vi "Coeficientes da norma - Não Uniforme.vi"(2 "Tipo de roseta":u16(ring) items=["Roseta A", "Roseta B", "Roseta C"], 3 "Diâmetro do furo":dbl, 4 "Diâmetro da roseta":dbl) -> (0 "Matrizes":T1, 1 "Vetor das medidas":dbl[](array[numeric]))   [LabVIEW 2016]
uses:
  <vilib>/Analysis/baseanly.llb/Real A x B.vi
  <vilib>/Analysis/NI_AALBase.lvlib
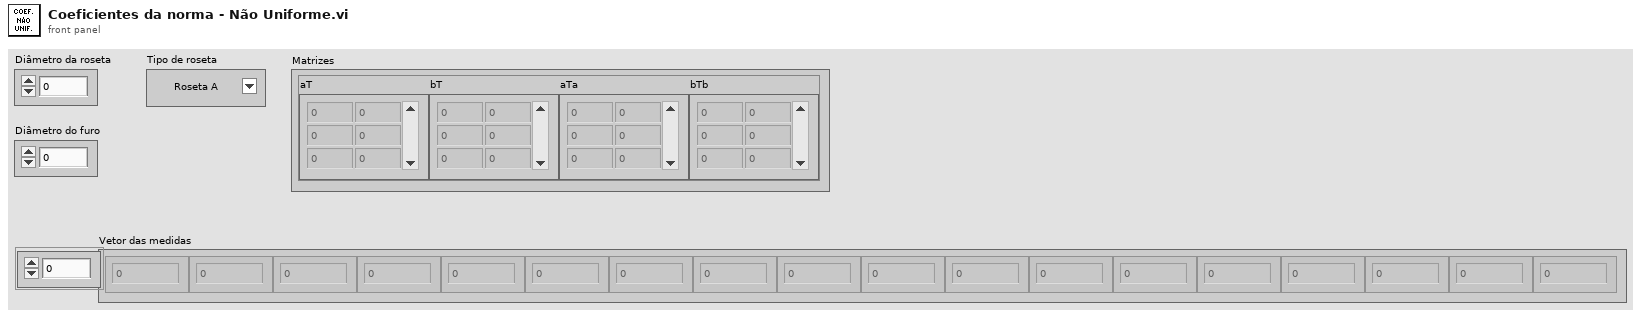
[diagram p1: front panel]
types:
  T1 = typedef "Matrizes não uniforme.ctl" = cluster{"aT":dbl[][], "bT":dbl[][], "aTa":dbl[][], "bTb":dbl[][]}
  T2 = typedef "NI_Matrix.lvlib/RealMatrix.ctl" = dbl[][]
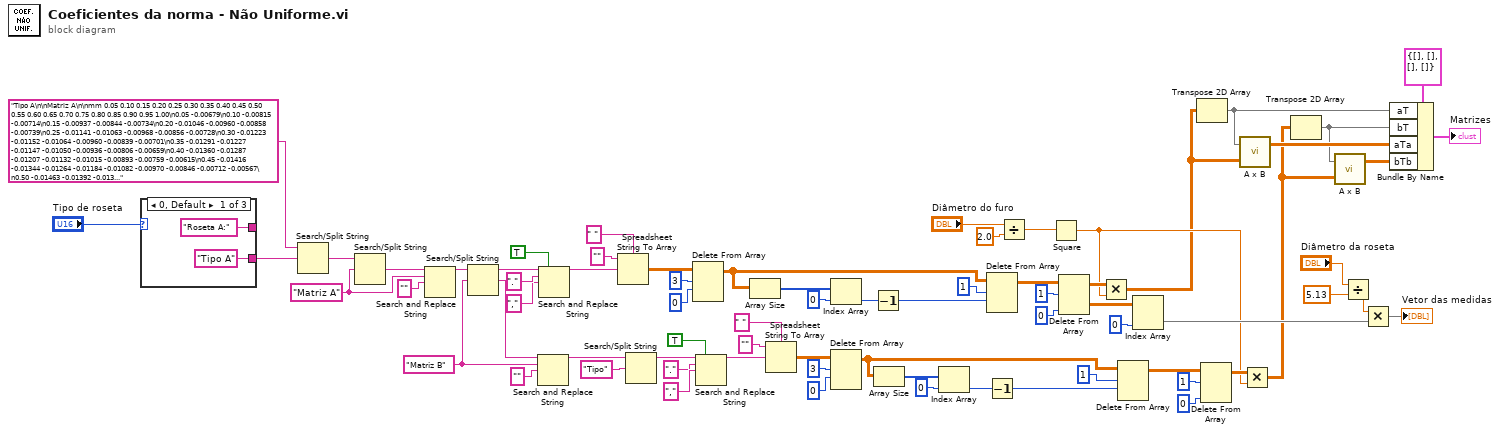
[diagram p0: block diagram]
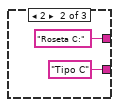
[diagram p2: hidden frame]
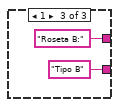
[diagram p3: hidden frame]
diagram:
  w44 = "Matriz B" ("search string/char (-)")
  w69 = "Matriz A" ("search string/char (-)")
  n1 = case shown="0, Default" "Tipo de roseta" {
    tunnel: ["Roseta A:" "Roseta C:" "Roseta B:"] -> _
    tunnel: ["Tipo A" "Tipo C" "Tipo B"] -> w21
    frame 0, Default {
    }
    frame 2 {
    }
    frame 1 {
    }
  }
  n2 = Search/Split String(string="Tipo A\n\nMatriz A\n\nmm 0.05 0.10 0.15 0.20 0.25 0.30 0.35 0.40 0.45 0.50 0.55 0.60 0.65 0.70 0.75 0.80 0.85 0.90 0.95 1.00\n0.05 -0.00679\n0.10 -0.00815 -0.00714\n0.15 -0.00937 -0.00844 -0.00734\n0.20 -0.01046 -0.00960 -0.00858 -0.00739\n0.25 -0.01141 -0.01063 -0.00968 -0.00856 -0.00728\n0.30 -0.01223 -0.01152 -0.01064 -0.00960 -0.00839 -0.00701\n0.35 -0.01291 -0.01227 -0.01147 -0.01050 -0.00936 -0.00806 -0.00659\n0.40 -0.01360 -0.01287 -0.01207 -0.01132 -0.01015 -0.00893 -0.00759 -0.00615\n0.45 -0.01416 -0.01344 -0.01264 -0.01184 -0.01082 -0.00970 -0.00846 -0.00712 -0.00567\n0.50 -0.01463 -0.01392 -0.01312 -0.01223 -0.01134 -0.01031 -0.00917 -0.00793 -0.00657 -0.00511\n0.55 -0.01508 -0.01434 -0.01354 -0.01270 -0.01173 -0.01072 -0.00977 -0.00854 -0.00730 -0.00600 -0.00464\n0.60 -0.01545 -0.01471 -0.01391 -0.01306 -0.01211 -0.01113 -0.01013 -0.00906 -0.00791 -0.00670 -0.00543 -0.00411\n0.65 -0.01578 -0.01503 -0.01422 -0.01340 -0.01243 -0.01146 -0.01049 -0.00938 -0.00842 -0.00722 -0.00604 -0.00485 -0.00364\n0.70 -0.01606 -0.01531 -0.01450 -0.01366 -0.01271 -0.01175 -0.01078 -0.00970 -0.00869 -0.00765 -0.00655 -0.00544 -0.00431 -0.00316\n0.75 -0.01629 -0.01554 -0.01473 -0.01390 -0.01294 -0.01199 -0.01102 -0.00996 -0.00892 -0.00795 -0.00693 -0.00589 -0.00484 -0.00378 -0.00270\n0.80 -0.01649 -0.01574 -0.01493 -0.01410 -0.01313 -0.01217 -0.01123 -0.01018 -0.00919 -0.00815 -0.00716 -0.00624 -0.00524 -0.00425 -0.00328 -0.00231\n0.85 -0.01665 -0.01590 -0.01510 -0.01426 -0.01330 -0.01234 -0.01138 -0.01036 -0.00938 -0.00836 -0.00738 -0.00644 -0.00555 -0.00464 -0.00373 -0.00283 -0.00195\n0.90 -0.01679 -0.01604 -0.01523 -0.01441 -0.01344 -0.01248 -0.01151 -0.01049 -0.00955 -0.00852 -0.00755 -0.00665 -0.00574 -0.00492 -0.00406 -0.00323 -0.00241 -0.00162\n0.95 -0.01692 -0.01617 -0.01536 -0.01452 -0.01357 -0.01261 -0.01164 -0.01063 -0.00967 -0.00866 -0.00770 -0.00679 -0.00592 -0.00508 -0.00432 -0.00353 -0.00277 -0.00203 -0.00131\n1.00 -0.01704 -0.01628 -0.01548 -0.01465 -0.01368 -0.01272 -0.01176 -0.01074 -0.00978 -0.00877 -0.00781 -0.00690 -0.00605 -0.00521 -0.00448 -0.00374 -0.00303 -0.00234 -0.00167 -0.00103\n\nMatriz B\n\nmm 0.05 0.10 0.15 0.20 0.25 0.30 0.35 0.40 0.45 0.50 0.55 0.60 0.65 0.70 0.75 0.80 0.85 0.90 0.95 1.00\n0.05 -0.01264\n0.10 -0.01470 -0.01352\n0.15 -0.01656 -0.01554 -0.01414\n0.20 -0.01821 -0.01735 -0.01611 -0.01449\n0.25 -0.01967 -0.01897 -0.01789 -0.01642 -0.01458\n0.30 -0.02092 -0.02038 -0.01946 -0.01815 -0.01647 -0.01439\n0.35 -0.02197 -0.02159 -0.02083 -0.01968 -0.01815 -0.01624 -0.01395\n0.40 -0.02308 -0.02256 -0.02182 -0.02112 -0.01952 -0.01778 -0.01576 -0.01348\n0.45 -0.02400 -0.02351 -0.02280 -0.02202 -0.02072 -0.01917 -0.01735 -0.01525 -0.01289\n0.50 -0.02481 -0.02434 -0.02366 -0.02273 -0.02167 -0.02031 -0.01868 -0.01678 -0.01460 -0.01216\n0.55 -0.02554 -0.02507 -0.02440 -0.02362 -0.02235 -0.02103 -0.01981 -0.01793 -0.01599 -0.01386 -0.01156\n0.60 -0.02616 -0.02571 -0.02505 -0.02428 -0.02305 -0.02177 -0.02045 -0.01890 -0.01715 -0.01522 -0.01310 -0.01081\n0.65 -0.02668 -0.02625 -0.02561 -0.02487 -0.02364 -0.02239 -0.02109 -0.01949 -0.01813 -0.01623 -0.01430 -0.01226 -0.01013\n0.70 -0.02715 -0.02673 -0.02611 -0.02536 -0.02417 -0.02294 -0.02164 -0.02012 -0.01866 -0.01708 -0.01531 -0.01345 -0.01149 -0.00944\n0.75 -0.02753 -0.02713 -0.02653 -0.02582 -0.02463 -0.02341 -0.02213 -0.02064 -0.01911 -0.01767 -0.01608 -0.01439 -0.01260 -0.01073 -0.00875\n0.80 -0.02789 -0.02749 -0.02690 -0.02620 -0.02502 -0.02382 -0.02256 -0.02108 -0.01968 -0.01807 -0.01652 -0.01511 -0.01344 -0.01172 -0.00995 -0.00812\n0.85 -0.02821 -0.02781 -0.02722 -0.02652 -0.02536 -0.02417 -0.02292 -0.02146 -0.02007 -0.01850 -0.01698 -0.01549 -0.01408 -0.01251 -0.01089 -0.00921 -0.00747\n0.90 -0.02848 -0.02809 -0.02750 -0.02682 -0.02565 -0.02447 -0.02324 -0.02176 -0.02041 -0.01885 -0.01736 -0.01590 -0.01441 -0.01312 -0.011591 -0.01004 -0.00847 -0.00688\n0.95 -0.02871 -0.02832 -0.02774 -0.02706 -0.02591 -0.02473 -0.02350 -0.02204 -0.02067 -0.01916 -0.01769 -0.01624 -0.01480 -0.01340 -0.01213 -0.01072 -0.00928 -0.00781 -0.00632\n1.00 -0.02889 -0.02851 -0.02794 -0.02727 -0.02612 -0.02495 -0.02373 -0.02227 -0.02089 -0.01940 -0.01796 -0.01655 -0.01511 -0.01367 -0.01249 -0.01121 -0.00989 -0.00856 -0.00719 -0.00581\n\nTipo B\n\nMatriz A\n\nmm 0.05 0.10 0.15 0.20 0.25 0.30 0.35 0.40 0.45 0.50 0.55 0.60 0.65 0.70 0.75 0.80 0.85 0.90 0.95 1.00\n0.05 -0.00726\n0.10 -0.00878 -0.00766\n0.15 -0.01013 -0.00909 -0.00788\n0.20 -0.01133 -0.01037 -0.00924 -0.00793\n0.25 -0.01237 -0.01149 -0.01043 -0.00921 -0.00781\n0.30 -0.01325 -0.01245 -0.01147 -0.01033 -0.00901 -0.00751\n0.35 -0.01397 -0.01325 -0.01235 -0.01129 -0.01004 -0.00863 -0.00704\n0.40 -0.01471 -0.01388 -0.01297 -0.01214 -0.01088 -0.00956 -0.00811 -0.00654\n0.45 -0.01533 -0.01450 -0.01360 -0.01268 -0.01161 -0.01039 -0.00904 -0.00758 -0.00599\n0.50 -0.01587 -0.01504 -0.01414 -0.01313 -0.01217 -0.01105 -0.00981 -0.00845 -0.00696 -0.00536\n0.55 -0.01634 -0.01550 -0.01460 -0.01367 -0.01257 -0.01147 -0.01046 -0.00909 -0.00774 -0.00633 -0.00486\n0.60 -0.01672 -0.01589 -0.01500 -0.01406 -0.01299 -0.01190 -0.01082 -0.00964 -0.00839 -0.00708 -0.00572 -0.00430\n0.65 -0.01705 -0.01621 -0.01532 -0.01441 -0.01332 -0.01225 -0.01118 -0.00997 -0.00892 -0.00764 -0.00637 -0.00509 -0.00379\n0.70 -0.01735 -0.01651 -0.01561 -0.01468 -0.01362 -0.01255 -0.01148 -0.01031 -0.00921 -0.00810 -0.00691 -0.00571 -0.00450 -0.00327\n0.75 -0.01759 -0.01675 -0.01586 -0.01493 -0.01387 -0.01280 -0.01174 -0.01059 -0.00945 -0.00840 -0.00730 -0.00619 -0.00506 -0.00392 -0.00277\n0.80 -0.01781 -0.01697 -0.01607 -0.01515 -0.01408 -0.01302 -0.01196 -0.01080 -0.00974 -0.00860 -0.00753 -0.00655 -0.00549 -0.00443 -0.00339 -0.00234\n0.85 -0.01799 -0.01715 -0.01625 -0.01533 -0.01426 -0.01320 -0.01213 -0.01099 -0.00992 -0.00881 -0.00775 -0.00674 -0.00581 -0.00484 -0.00387 -0.00291 -0.00195\n0.90 -0.01814 -0.01730 -0.01640 -0.01550 -0.01441 -0.01334 -0.01229 -0.01114 -0.01008 -0.00897 -0.00793 -0.00695 -0.00598 -0.00514 -0.00423 -0.00333 -0.00246 -0.00162\n0.95 -0.01829 -0.01744 -0.01654 -0.01561 -0.01454 -0.01347 -0.01242 -0.01129 -0.01021 -0.00912 -0.00809 -0.00710 -0.00617 -0.00528 -0.00449 -0.00366 -0.00285 -0.00207 -0.00131\n1.00 -0.01843 -0.01757 -0.01666 -0.01573 -0.01465 -0.01358 -0.01253 -0.01140 -0.01035 -0.00925 -0.00822 -0.00724 -0.00632 -0.00541 -0.00466 -0.00389 -0.00314 -0.00242 -0.00172 -0.00104\n\nMatriz B\n\nmm 0.05 0.10 0.15 0.20 0.25 0.30 0.35 0.40 0.45 0.50 0.55 0.60 0.65 0.70 0.75 0.80 0.85 0.90 0.95 1.00\n0.05 -0.01417\n0.10 -0.01653 -0.01516\n0.15 -0.01866 -0.01746 -0.01585\n0.20 -0.02055 -0.01953 -0.01810 -0.01624\n0.25 -0.02222 -0.02138 -0.02012 -0.01844 -0.01634\n0.30 -0.02365 -0.02299 -0.02190 -0.02040 -0.01848 -0.01614\n0.35 -0.02485 -0.02437 -0.02346 -0.02214 -0.02039 -0.01823 -0.01564\n0.40 -0.02610 -0.02547 -0.02459 -0.02375 -0.02195 -0.01997 -0.01769 -0.01510\n0.45 -0.02715 -0.02656 -0.02571 -0.02479 -0.02331 -0.02154 -0.01947 -0.01709 -0.01440\n0.50 -0.02806 -0.02750 -0.02670 -0.02561 -0.02440 -0.02283 -0.02097 -0.01879 -0.01631 -0.01353\n0.55 -0.02888 -0.02833 -0.02755 -0.02664 -0.02517 -0.02365 -0.02225 -0.02008 -0.01787 -0.01546 -0.01285\n0.60 -0.02958 -0.02906 -0.02830 -0.02740 -0.02598 -0.02450 -0.02298 -0.02119 -0.01919 -0.01699 -0.01460 -0.01202\n0.65 -0.03019 -0.02968 -0.02894 -0.02808 -0.02666 -0.02521 -0.02370 -0.02186 -0.02030 -0.01816 -0.01596 -0.01367 -0.01126\n0.70 -0.03072 -0.03023 -0.02950 -0.02864 -0.02727 -0.02584 -0.02435 -0.02257 -0.02089 -0.01910 -0.01710 -0.01499 -0.01278 -0.01046\n0.75 -0.03116 -0.03068 -0.02998 -0.02914 -0.02778 -0.02638 -0.02491 -0.02316 -0.02139 -0.01976 -0.01795 -0.01603 -0.01401 -0.01188 -0.00964\n0.80 -0.03158 -0.03108 -0.03038 -0.02956 -0.02822 -0.02684 -0.02539 -0.02366 -0.02202 -0.02022 -0.01846 -0.01685 -0.01493 -0.01299 -0.01100 -0.00895\n0.85 -0.03192 -0.03143 -0.03073 -0.02990 -0.02859 -0.02723 -0.02580 -0.02410 -0.02247 -0.02071 -0.01899 -0.01729 -0.01567 -0.01390 -0.01207 -0.01019 -0.00825\n0.90 -0.03221 -0.03173 -0.03104 -0.03022 -0.02891 -0.02756 -0.02616 -0.02444 -0.02287 -0.02112 -0.01942 -0.01779 -0.01608 -0.01459 -0.01288 -0.01115 -0.00940 -0.00762\n0.95 -0.03247 -0.03200 -0.03131 -0.03048 -0.02919 -0.02785 -0.02645 -0.02475 -0.02317 -0.02146 -0.01979 -0.01817 -0.01650 -0.01493 -0.01349 -0.01191 -0.01030 -0.00866 -0.00700\n1.00 -0.03268 -0.03222 -0.03154 -0.03074 -0.02944 -0.02810 -0.02671 -0.02501 -0.02342 -0.02173 -0.02008 -0.01848 -0.01684 -0.01521 -0.01389 -0.01245 -0.01098 -0.00948 -0.00796 -0.00641\n\nTipo C\n\nMatriz A\n\nmm 0.05 0.10 0.15 0.20 0.25 0.30 0.35 0.40 0.45 0.50 0.55 0.60 0.65 0.70 0.75 0.80 0.85 0.90 0.95 1.00 1.05 1.10 1.15 1.20 1.25\n0.05 -0.01704\n0.10 -0.02009 -0.01741\n0.15 -0.02285 -0.02043 -0.01749\n0.20 -0.02531 -0.02315 -0.02047 -0.01730\n0.25 -0.02748 -0.02557 -0.02316 -0.02024 -0.01681\n0.30 -0.02945 -0.02757 -0.02547 -0.02310 -0.01965 -0.01608\n0.35 -0.03124 -0.02938 -0.02730 -0.02526 -0.02212 -0.01885 -0.01523\n0.40 -0.03282 -0.03092 -0.02886 -0.02668 -0.02402 -0.02133 -0.01775 -0.01417\n0.45 -0.03422 -0.03230 -0.03023 -0.02806 -0.02549 -0.02306 -0.01988 -0.01659 -0.01307\n0.50 -0.03545 -0.03347 -0.03137 -0.02921 -0.02669 -0.02422 -0.02148 -0.01867 -0.01521 -0.01192\n0.55 -0.03649 -0.03451 -0.03241 -0.03020 -0.02774 -0.02530 -0.02269 -0.02012 -0.01695 -0.01386 -0.01074\n0.60 -0.03735 -0.03534 -0.03324 -0.03108 -0.02865 -0.02621 -0.02370 -0.02123 -0.01824 -0.01546 -0.01243 -0.00949\n0.65 -0.03810 -0.03609 -0.03399 -0.03178 -0.02942 -0.02700 -0.02448 -0.02212 -0.01926 -0.01661 -0.01385 -0.01110 -0.00835\n0.70 -0.03872 -0.03672 -0.03461 -0.03241 -0.03006 -0.02771 -0.02510 -0.02268 -0.02005 -0.01753 -0.01492 -0.01248 -0.00983 -0.00728\n0.75 -0.03927 -0.03727 -0.03516 -0.03293 -0.03059 -0.02826 -0.02568 -0.02320 -0.02064 -0.01823 -0.01572 -0.01344 -0.01102 -0.00864 -0.00630\n0.80 -0.03972 -0.03772 -0.03563 -0.03343 -0.03101 -0.02869 -0.02615 -0.02371 -0.02117 -0.01877 -0.01633 -0.01408 -0.01185 -0.00978 -0.00753 -0.00540\n0.85 -0.04014 -0.03811 -0.03600 -0.03382 -0.03141 -0.02905 -0.02654 -0.02411 -0.02161 -0.01924 -0.01682 -0.01461 -0.01246 -0.01052 -0.00851 -0.00653 -0.00456\n0.90 -0.04050 -0.03845 -0.03632 -0.03412 -0.03173 -0.02935 -0.02688 -0.02445 -0.02198 -0.01964 -0.01724 -0.01501 -0.01296 -0.01100 -0.00924 -0.00742 -0.00561 -0.00381\n0.95 -0.04083 -0.03874 -0.03658 -0.03436 -0.03199 -0.02960 -0.02712 -0.02477 -0.02230 -0.01996 -0.01756 -0.01540 -0.01334 -0.01142 -0.00968 -0.00810 -0.00639 -0.00476 -0.00317\n1.00 -0.04110 -0.03899 -0.03682 -0.03458 -0.03223 -0.02983 -0.02735 -0.02497 -0.02256 -0.02024 -0.01785 -0.01567 -0.01366 -0.01175 -0.01008 -0.00849 -0.00699 -0.00547 -0.00401 -0.00259\n1.05 -0.04131 -0.03920 -0.03702 -0.03477 -0.03244 -0.03010 -0.02756 -0.02513 -0.02274 -0.02048 -0.01808 -0.01589 -0.01388 -0.01204 -0.01037 -0.00883 -0.00733 -0.00596 -0.00468 -0.00335 -0.00210\n1.10 -0.04149 -0.03938 -0.03720 -0.03493 -0.03262 -0.03028 -0.02775 -0.02531 -0.02290 -0.02064 -0.01828 -0.01609 -0.01410 -0.01224 -0.01062 -0.00909 -0.00765 -0.00631 -0.00511 -0.00392 -0.00278 -0.00168\n1.15 -0.04162 -0.03952 -0.03734 -0.03509 -0.03275 -0.03043 -0.02790 -0.02548 -0.02306 -0.02077 -0.01843 -0.01631 -0.01429 -0.01242 -0.01081 -0.00932 -0.00788 -0.00658 -0.00541 -0.00434 -0.00331 -0.00230 -0.00137\n1.20 -0.04175 -0.03965 -0.03748 -0.03521 -0.03287 -0.03054 -0.02802 -0.02561 -0.02320 -0.02091 -0.01855 -0.01643 -0.01444 -0.01258 -0.01098 -0.00949 -0.00807 -0.00679 -0.00565 -0.00463 -0.00367 -0.00275 -0.00188 -0.00105\n1.25 -0.04188 -0.03977 -0.03759 -0.03535 -0.03298 -0.03061 -0.02811 -0.02572 -0.02330 -0.02103 -0.01865 -0.01652 -0.01455 -0.01271 -0.01111 -0.00964 -0.00822 -0.00695 -0.00581 -0.00485 -0.00393 -0.00304 -0.00227 -0.00151 -0.00076\n\nMatriz B\n\nmm 0.05 0.10 0.15 0.20 0.25 0.30 0.35 0.40 0.45 0.50 0.55 0.60 0.65 0.70 0.75 0.80 0.85 0.90 0.95 1.00 1.05 1.10 1.15 1.20 1.25\n0.05 -0.02533\n0.10 -0.02958 -0.02675\n0.15 -0.03345 -0.03109 -0.02767\n0.20 -0.03693 -0.03504 -0.03209 -0.02808\n0.25 -0.04004 -0.03862 -0.03614 -0.03259 -0.02798\n0.30 -0.04292 -0.04164 -0.03970 -0.03704 -0.03244 -0.02744\n0.35 -0.04555 -0.04439 -0.04258 -0.04050 -0.03641 -0.03194 -0.02670\n0.40 -0.04790 -0.04676 -0.04511 -0.04293 -0.03961 -0.03607 -0.03095 -0.02563\n0.45 -0.05005 -0.04892 -0.04728 -0.04526 -0.04211 -0.03909 -0.03458 -0.02976 -0.02442\n0.50 -0.05200 -0.05084 -0.04918 -0.04711 -0.04419 -0.04115 -0.03730 -0.03340 -0.02817 -0.02304\n0.55 -0.05363 -0.05253 -0.05092 -0.04881 -0.04599 -0.04307 -0.03955 -0.03601 -0.03129 -0.02654 -0.02155\n0.60 -0.05495 -0.05391 -0.05237 -0.05036 -0.04758 -0.04467 -0.04136 -0.03798 -0.03362 -0.02952 -0.02466 -0.01984\n0.65 -0.05614 -0.05513 -0.05362 -0.05164 -0.04893 -0.04609 -0.04280 -0.03962 -0.03548 -0.03163 -0.02733 -0.02289 -0.01827\n0.70 -0.05714 -0.05615 -0.05469 -0.05276 -0.05007 -0.04730 -0.04397 -0.04076 -0.03696 -0.03326 -0.02935 -0.02559 -0.02113 -0.01677\n0.75 -0.05804 -0.05706 -0.05560 -0.05371 -0.05105 -0.04829 -0.04503 -0.04179 -0.03811 -0.03461 -0.03085 -0.02745 -0.02345 -0.01944 -0.01536\n0.80 -0.05882 -0.05782 -0.05635 -0.05448 -0.05186 -0.04915 -0.04590 -0.04273 -0.03912 -0.03565 -0.03202 -0.02862 -0.02506 -0.02168 -0.01784 -0.01406\n0.85 -0.05949 -0.05850 -0.05704 -0.05514 -0.05255 -0.04985 -0.04664 -0.04350 -0.03996 -0.03657 -0.03300 -0.02966 -0.02624 -0.02314 -0.1978 -0.01633 -0.01275\n0.90 -0.06006 -0.05908 -0.05762 -0.05571 -0.05315 -0.05044 -0.04727 -0.04412 -0.04068 -0.03734 -0.03382 -0.03048 -0.02723 -0.02407 -0.02126 -0.01813 -0.01487 -0.01149\n0.95 -0.06051 -0.05955 -0.05811 -0.05622 -0.05364 -0.05100 -0.04781 -0.04465 -0.04125 -0.03799 -0.03448 -0.03124 -0.02799 -0.02494 -0.02211 -0.01956 -0.01647 -0.01341 -0.01034\n1.00 -0.06091 -0.05997 -0.05854 -0.05664 -0.05407 -0.05142 -0.04828 -0.04513 -0.04176 -0.03850 -0.03505 -0.03182 -0.02864 -0.02561 -0.02290 -0.02031 -0.01771 -0.01495 -0.01216 -0.00935\n1.05 -0.06124 -0.06030 -0.05888 -0.05703 -0.05444 -0.05175 -0.04865 -0.04559 -0.04218 -0.03895 -0.03550 -0.03229 -0.02915 -0.02620 -0.02348 -0.02095 -0.01842 -0.01600 -0.01363 -0.01102 -0.00854\n1.10 -0.06153 -0.06059 -0.05918 -0.05733 -0.05478 -0.05208 -0.04898 -0.04592 -0.04254 -0.03932 -0.03590 -0.03269 -0.02961 -0.02666 -0.02400 -0.02146 -0.01908 -0.01675 -0.01459 -0.01227 -0.01000 -0.00775\n1.15 -0.06175 -0.06083 -0.05943 -0.05757 -0.05505 -0.05243 -0.04927 -0.04618 -0.04282 -0.03962 -0.03623 -0.03308 -0.02999 -0.02710 -0.02444 -0.02191 -0.01955 -0.01733 -0.01523 -0.01311 -0.01116 -0.00907 -0.00703\n1.20 -0.06195 -0.06104 -0.05965 -0.05779 -0.05528 -0.05267 -0.04953 -0.04644 -0.04308 -0.03986 -0.03650 -0.03337 -0.03030 -0.02743 -0.02480 -0.02229 -0.01996 -0.01776 -0.01576 -0.01373 -0.01191 -0.01010 -0.00824 -0.00637\n1.25 -0.06211 -0.06122 -0.05984 -0.05801 -0.05547 -0.05285 -0.04972 -0.04667 -0.04331 -0.04009 -0.03674 -0.03361 -0.03055 -0.02770 -0.02507 -0.02263 -0.02028 -0.01810 -0.01609 -0.01420 -0.01241 -0.01081 -0.00926 -0.00751 -0.00582\n", search string/char (-)=w21) -> (match + rest of string=w72:string)  [unwired: 1 in, 2 out]
  n3 = Search/Split String(string=w72, search string/char (-)=w69) -> (match + rest of string=w70:string)  [unwired: 1 in, 2 out]
  n4 = Search and Replace String(input string=w70, search string=w69, replace string="" ("replace string (\"\")")) -> (result string=w68:string)  [unwired: 5 in, 3 out]
  n5 = Search/Split String(string=w68, search string/char (-)=w44) -> (substring before match=w62:string, match + rest of string=w45:string)  [unwired: 1 in, 1 out]
  n6 = Search and Replace String(input string=w45, search string=w44, replace string="" ("replace string (\"\")")) -> (result string=w43:string)  [unwired: 5 in, 3 out]
  n7 = Search and Replace String(replace all?=TRUE ("replace all? (F)"), input string=w62, search string=".", replace string="," ("replace string (\"\")")) -> (result string=w67:string)  [unwired: 4 in, 3 out]
  n8 = Spreadsheet String To Array(delimiter (Tab)=" ", format string="", spreadsheet string=w67) -> (array=w58:dbl[][])  [unwired: 1 in]
  n9 = Search/Split String(string=w43, search string/char (-)="Tipo") -> (substring before match=w24:string)  [unwired: 1 in, 2 out]
  n10 = Delete From Array(array=w58, length=3, index (row)=0) -> (array with subset deleted=w51:dbl[][])  [unwired: 1 in, 1 out]
  n11 = Search and Replace String(replace all?=TRUE ("replace all? (F)"), input string=w24, search string=".", replace string="," ("replace string (\"\")")) -> (result string=w23:string)  [unwired: 4 in, 3 out]
  n12 = Array Size(array=w51) -> (size(s)=w49:i32[])
  n13 = Spreadsheet String To Array(delimiter (Tab)=" ", format string="", spreadsheet string=w23) -> (array=w32:dbl[][])  [unwired: 1 in]
  n14 = Index Array(array=w49, index=0 ("disabled index (col)")) -> (element=w48:i32)
  n15 = Delete From Array(array=w32, length=3, index (row)=0) -> (array with subset deleted=w37:dbl[][])  [unwired: 1 in, 1 out]
  n16 = Decrement(x=w48) -> (x-1=w47:i32)
  n17 = Array Size(array=w37) -> (size(s)=w39:i32[])
  n18 = Index Array(array=w39, index=0 ("disabled index (col)")) -> (element=w40:i32)
  n19 = Delete From Array(array=w51, length=1, index (row)=w47) -> (array with subset deleted=w52:dbl[][])  [unwired: 1 in, 1 out]
  n20 = Decrement(x=w40) -> (x-1=w41:i32)
  n21 = Divide(x="Diâmetro do furo", y=2.0) -> (x/y=w12:dbl)
  n22 = Square(x=w12) -> (x^2=w9:dbl)
  n23 = Delete From Array(array=w52, length=1, index (col)=0 ("index (row)")) -> (deleted portion=w55:dbl[][], array with subset deleted=w11:dbl[][])  [unwired: 1 in]
  n24 = Multiply(x=w11, y=w9) -> (x*y=w1:dbl[][])
  n25 = Delete From Array(array=w37, length=1, index (row)=w41) -> (array with subset deleted=w36:dbl[][])  [unwired: 1 in, 1 out]
  n26 = Index Array(array=w55, index (col)=0 ("disabled index (col)")) -> (element=w17:dbl[])  [unwired: 1 in]
  n27 = Transpose 2D Array(2D array=w1) -> (transposed array=w2:dbl[][])
  n28 = Delete From Array(array=w36, length=1, index (col)=0 ("index (row)")) -> (array with subset deleted=w10:dbl[][])  [unwired: 1 in, 1 out]
  n29 = call-poly <vilib>:"A x B.vi"("B"=w1, "A"=w2) -> ("A x B"=w6:T2)  [unwired: 1 out]
  n30 = Multiply(x=w10, y=w9) -> (x*y=w4:dbl[][])
  n31 = Transpose 2D Array(2D array=w4) -> (transposed array=w5:dbl[][])
  n32 = call-poly <vilib>:"A x B.vi"("B"=w4, "A"=w5) -> ("A x B"=w3:T2)  [unwired: 1 out]
  n33 = Divide(x="Diâmetro da roseta", y=5.13) -> (x/y=w16:dbl)
  n34 = Multiply(x=w16, y=w17) -> (x*y=→"Vetor das medidas":dbl[])
  n35 = Bundle By Name(cluster=T1 {"aT"=[], "bT"=[], "aTa"=[], "bTb"=[]} ("Matrizes não uniforme"), "aT"=w2, "bT"=w5, "aTa"=w6, "bTb"=w3) -> (→"Matrizes":T1)
